vi "Modles Value Change.vi"(8 "UI":refnum<queue>, 10 "New Modules":T1={"Module01"={"Names"={"Module Name"="", "Set Value"="", "Real Value"="", "FB Value"="", "Unit"="", "Identifier"="", "IdentifierW"="写入标识符", "Decimal"="位数", "AS"=FALSE, "AR"=FALSE, "Con"=FALSE}, "Data"=[], "Digit"=0.0}, "Module02"={"Names"={"Module Name"="", "Set Value"="", "Real Value"="", "FB Value"="", "Unit"="", "Identifier"="", "IdentifierW"="写入标识符", "Decimal"="位数", "AS"=FALSE, "AR"=FALSE, "Con"=FALSE}, "Data"=[], "Digit"=0.0}, "Module03"={"Names"={"Module Name"="", "Set Value"="", "Real Value"="", "FB Value"="", "Unit"="", "Identifier"="", "IdentifierW"="写入标识符", "Decimal"="位数", "AS"=FALSE, "AR"=FALSE, "Con"=FALSE}, "Data"=[], "Digit"=0.0}, "Module04"={"Names"={"Module Name"="", "Set Value"="", "Real Value"="", "FB Value"="", "Unit"="", "Identifier"="", "IdentifierW"="写入标识符", "Decimal"="位数", "AS"=FALSE, "AR"=FALSE, "Con"=FALSE}, "Data"=[], "Digit"=0.0}, "Module05"={"Names"={"Module Name"="", "Set Value"="", "Real Value"="", "FB Value"="", "Unit"="", "Identifier"="", "IdentifierW"="写入标识符", "Decimal"="位数", "AS"=FALSE, "AR"=FALSE, "Con"=FALSE}, "Data"=[], "Digit"=0.0}, "Module06"={"Names"={"Module Name"="", "Set Value"="", "Real Value"="", "FB Value"="", "Unit"="", "Identifier"="", "IdentifierW"="写入标识符", "Decimal"="位数", "AS"=FALSE, "AR"=FALSE, "Con"=FALSE}, "Data"=[], "Digit"=0.0}, "Module07"={"Names"={"Module Name"="", "Set Value"="", "Real Value"="", "FB Value"="", "Unit"="", "Identifier"="", "IdentifierW"="写入标识符", "Decimal"="位数", "AS"=FALSE, "AR"=FALSE, "Con"=FALSE}, "Data"=[], "Digit"=0.0}, "Module08"={"Names"={"Module Name"="", "Set Value"="", "Real Value"="", "FB Value"="", "Unit"="", "Identifier"="", "IdentifierW"="写入标识符", "Decimal"="位数", "AS"=FALSE, "AR"=FALSE, "Con"=FALSE}, "Data"=[], "Digit"=0.0}, "Module09"={"Names"={"Module Name"="", "Set Value"="", "Real Value"="", "FB Value"="", "Unit"="", "Identifier"="", "IdentifierW"="写入标识符", "Decimal"="位数", "AS"=FALSE, "AR"=FALSE, "Con"=FALSE}, "Data"=[], "Digit"=0.0}, "Module10"={"Names"={"Module Name"="", "Set Value"="", "Real Value"="", "FB Value"="", "Unit"="", "Identifier"="", "IdentifierW"="写入标识符", "Decimal"="位数", "AS"=FALSE, "AR"=FALSE, "Con"=FALSE}, "Data"=[], "Digit"=0.0}, "Module11"={"Names"={"Module Name"="", "Set Value"="", "Real Value"="", "FB Value"="", "Unit"="", "Identifier"="", "IdentifierW"="写入标识符", "Decimal"="位数", "AS"=FALSE, "AR"=FALSE, "Con"=FALSE}, "Data"=[], "Digit"=0.0}}, 11 "Old Modules":T1={"Module01"={"Names"={"Module Name"="", "Set Value"="", "Real Value"="", "FB Value"="", "Unit"="", "Identifier"="", "IdentifierW"="写入标识符", "Decimal"="位数", "AS"=FALSE, "AR"=FALSE, "Con"=FALSE}, "Data"=[], "Digit"=0.0}, "Module02"={"Names"={"Module Name"="", "Set Value"="", "Real Value"="", "FB Value"="", "Unit"="", "Identifier"="", "IdentifierW"="写入标识符", "Decimal"="位数", "AS"=FALSE, "AR"=FALSE, "Con"=FALSE}, "Data"=[], "Digit"=0.0}, "Module03"={"Names"={"Module Name"="", "Set Value"="", "Real Value"="", "FB Value"="", "Unit"="", "Identifier"="", "IdentifierW"="写入标识符", "Decimal"="位数", "AS"=FALSE, "AR"=FALSE, "Con"=FALSE}, "Data"=[], "Digit"=0.0}, "Module04"={"Names"={"Module Name"="", "Set Value"="", "Real Value"="", "FB Value"="", "Unit"="", "Identifier"="", "IdentifierW"="写入标识符", "Decimal"="位数", "AS"=FALSE, "AR"=FALSE, "Con"=FALSE}, "Data"=[], "Digit"=0.0}, "Module05"={"Names"={"Module Name"="", "Set Value"="", "Real Value"="", "FB Value"="", "Unit"="", "Identifier"="", "IdentifierW"="写入标识符", "Decimal"="位数", "AS"=FALSE, "AR"=FALSE, "Con"=FALSE}, "Data"=[], "Digit"=0.0}, "Module06"={"Names"={"Module Name"="", "Set Value"="", "Real Value"="", "FB Value"="", "Unit"="", "Identifier"="", "IdentifierW"="写入标识符", "Decimal"="位数", "AS"=FALSE, "AR"=FALSE, "Con"=FALSE}, "Data"=[], "Digit"=0.0}, "Module07"={"Names"={"Module Name"="", "Set Value"="", "Real Value"="", "FB Value"="", "Unit"="", "Identifier"="", "IdentifierW"="写入标识符", "Decimal"="位数", "AS"=FALSE, "AR"=FALSE, "Con"=FALSE}, "Data"=[], "Digit"=0.0}, "Module08"={"Names"={"Module Name"="", "Set Value"="", "Real Value"="", "FB Value"="", "Unit"="", "Identifier"="", "IdentifierW"="写入标识符", "Decimal"="位数", "AS"=FALSE, "AR"=FALSE, "Con"=FALSE}, "Data"=[], "Digit"=0.0}, "Module09"={"Names"={"Module Name"="", "Set Value"="", "Real Value"="", "FB Value"="", "Unit"="", "Identifier"="", "IdentifierW"="写入标识符", "Decimal"="位数", "AS"=FALSE, "AR"=FALSE, "Con"=FALSE}, "Data"=[], "Digit"=0.0}, "Module10"={"Names"={"Module Name"="", "Set Value"="", "Real Value"="", "FB Value"="", "Unit"="", "Identifier"="", "IdentifierW"="写入标识符", "Decimal"="位数", "AS"=FALSE, "AR"=FALSE, "Con"=FALSE}, "Data"=[], "Digit"=0.0}, "Module11"={"Names"={"Module Name"="", "Set Value"="", "Real Value"="", "FB Value"="", "Unit"="", "Identifier"="", "IdentifierW"="写入标识符", "Decimal"="位数", "AS"=FALSE, "AR"=FALSE, "Con"=FALSE}, "Data"=[], "Digit"=0.0}}) -> ()   [LabVIEW 2020]
uses:
  0007 Controls/Data Element Single.ctl
  0007 Controls/Data Modules.ctl
  0007 Controls/Data Module.ctl
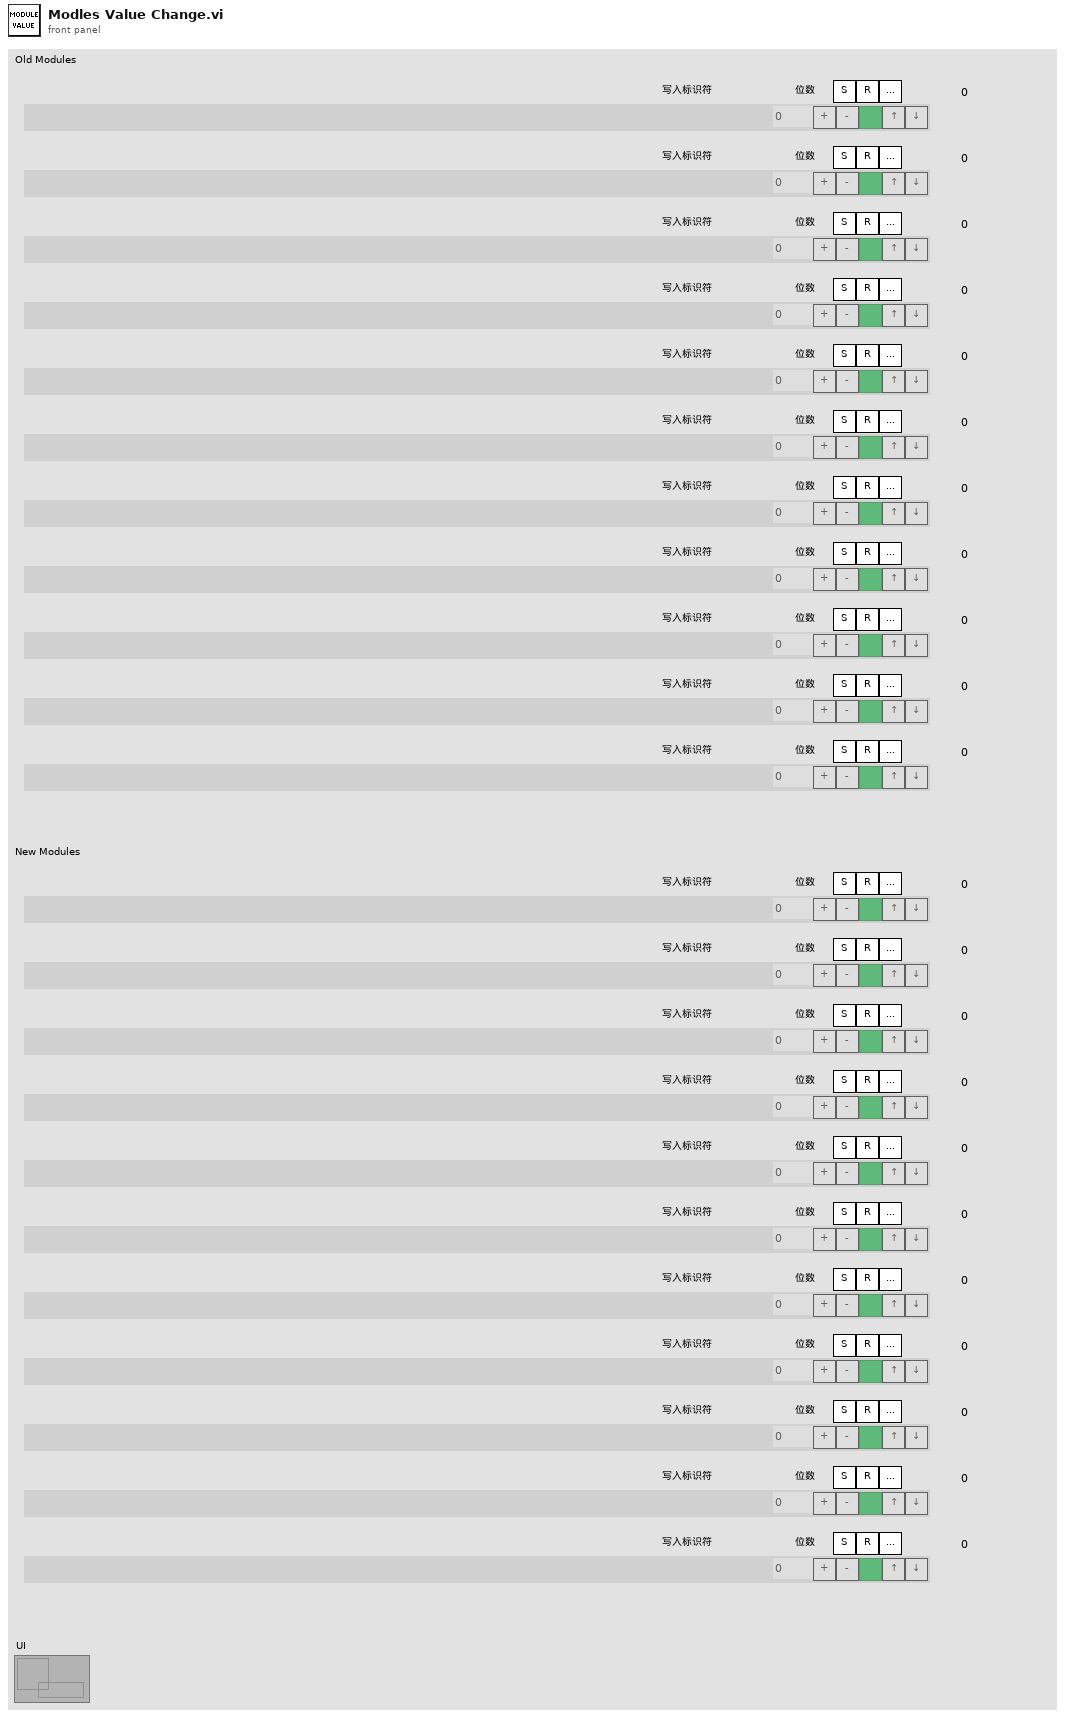
[diagram p1: front panel]
types:
  T1 = typedef "Data Module.ctl" = cluster{"Module01":T2, "Module02":T2, "Module03":T2, "Module04":T2, "Module05":T2, "Module06":T2, "Module07":T2, "Module08":T2, "Module09":T2, "Module10":T2, "Module11":T2}
  T2 = typedef "Data Modules.ctl" = cluster{"Names":cluster{"Module Name":string, "Set Value":string, "Real Value":string, "FB Value":string, "Unit":string, "Identifier":string, "IdentifierW":string, "Decimal":string, "AS":bool, "AR":bool, "Con":bool}, "Data":T3[], "Digit":dbl}
  T3 = typedef "Data Element Single.ctl" = cluster{"Name":string, "Set Value":string, "Real Value":string, "FB Value":string, "Unit":string, "Identifier":string, "Write Name":string, "Decimal":u16, "AS":bool, "AR":bool, "ALM":bool, "Up":bool, "Down":bool}
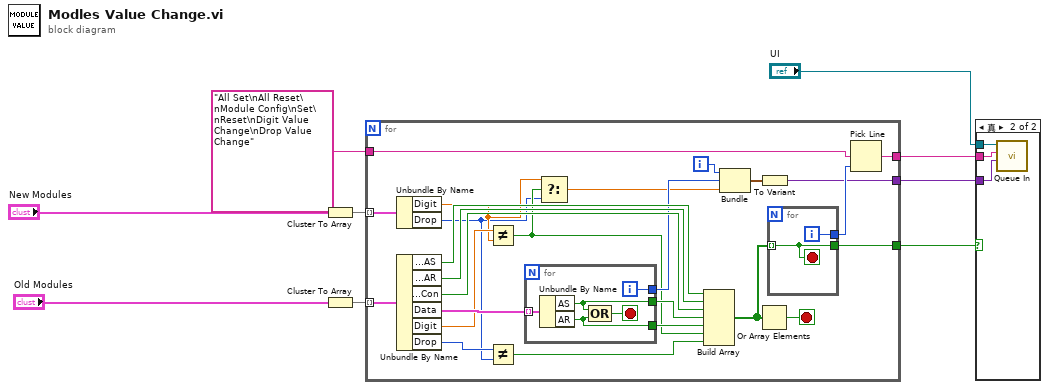
[diagram p0: block diagram]
diagram:
  n1 = Cluster To Array(cluster="New Modules") -> (array=w6:T2[])
  n2 = Cluster To Array(cluster="Old Modules") -> (array=w9:T2[])
  n3 = for {
    tunnel: w9 -> [w34] mode=indexing
    tunnel: [w19] -> w8
    tunnel: w6 -> [w26] mode=indexing
    tunnel: "All Set\nAll Reset\nModule Config\nSet\nReset\nDigit Value Change\nDrop Value Change" ("Message") -> [w21]
    tunnel: [w18] -> w2
    tunnel: [w14] -> w1
    i -> [w16]
    stop <- w27 stop-if-true
    n4 = Unbundle By Name(w26) -> ("Digit"=w12:dbl, "Drop"=w11:u16)
    n5 = Unbundle By Name(w34) -> ("Names.AS"=w22:bool, "Names.AR"=w32:bool, "Names.Con"=w31:bool, "Data"=w33:T3[], "Digit"=w24:dbl, "Drop"=w23:u16)
    n6 = Not Equal?(x=w24, y=w12) -> (x != y?=w13:bool)
    n7 = Not Equal?(x=w23, y=w11) -> (x != y?=w25:bool)
    n8 = for {
      tunnel: w33 -> [w41] mode=indexing
      tunnel: [w39] -> w30
      tunnel: [w38] -> w29
      tunnel: [w37] -> w15
      i -> [w37]
      stop <- w40 stop-if-true
      n9 = Unbundle By Name(w41) -> ("AS"=w39:bool, "AR"=w38:bool)
      n10 = Compound Arithmetic op=OR ("复合运算")(w39, w38) -> (w40:bool)
    }
    n11 = Select(t=w12, s=w13, f=w11) -> (s? t:f=w10:dbl)
    n12 = Build Array(w22, w32, w31, w30, w29, w13, w25) -> (w28:bool[])
    n13 = Bundle(w16, w15, "Digit"=w10) -> (w17:cluster{i32, i32, "Digit":dbl})  [unwired: 1 in]
    n14 = Or Array Elements(Boolean array=w28) -> (logical OR=w27:bool)
    n15 = To Variant(anything=w17) -> (Variant=w14:variant)
    n16 = for {
      tunnel: w28 -> [w35] mode=indexing
      tunnel: [w36] -> w20
      tunnel: [w35] -> w19
      i -> [w36]
      stop <- w35 stop-if-true
    }
    n17 = Pick Line(multi-line string=w21, line index=w20) -> (output string=w18:string)  [unwired: 1 in]
  }
  n18 = case shown="真" w8 {
    tunnel: "UI" -> [_ w44]
    tunnel: w2 -> [_ w43]
    tunnel: w1 -> [_ w42]
    frame False {
    }
    frame True {
      n19 = call "Queue In.vi"("Data"=w42, "Message"=w43, "Queue In"=w44) -> ()  [unwired: 7 in, 2 out]
    }
  }
